vi "MultiAxisPositioningWithTime.vi"(6 "error in":errorcluster, 8 "Input_Cluster":T1, 9 "connection ID":refnum<k5>) -> (0 "error out":errorcluster, 2 "return":T2, 3 "connection ID":refnum<k5>)   [LabVIEW 2016, in "AMC_VIs.lvlib"]
doc: "Simultaneously set 3 axes positions\n and get positions to minimize network latency"
uses:
  AMC_VIs.lvlib
panel:
  out "params_cluster":T3
  in  "Params_cluster":T4
  in  "results_cluster":T5
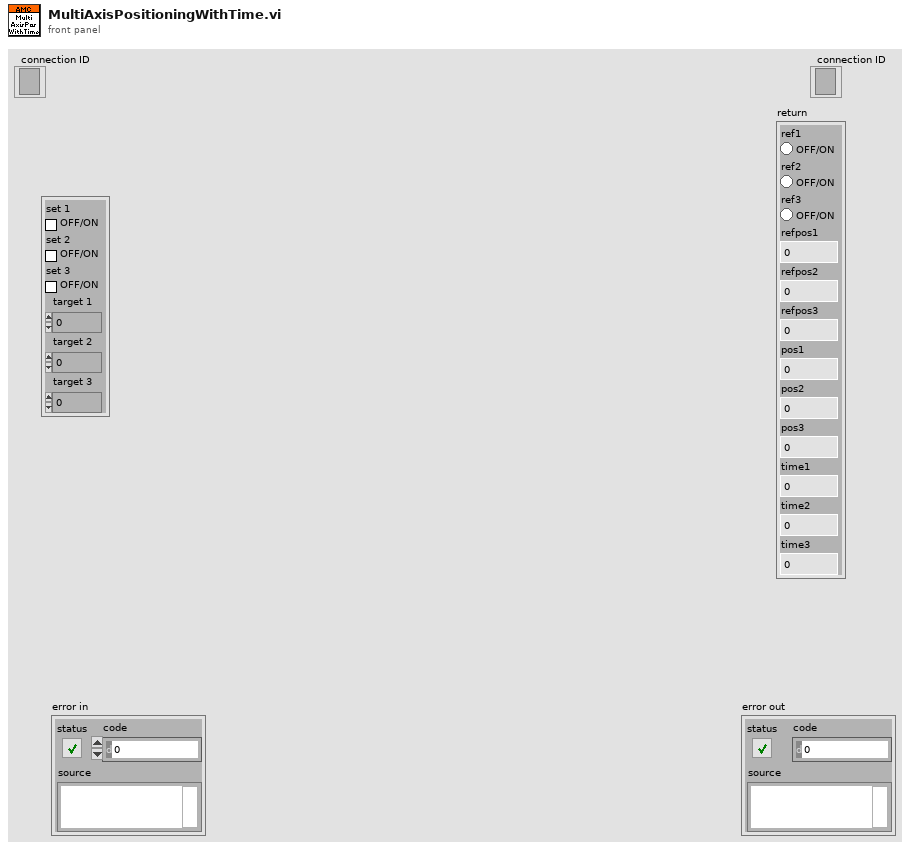
[diagram p1: front panel]
types:
  T1 = cluster{"set 1":bool, "set 2":bool, "set 3":bool, "target 1":i32, "target 2":i32, "target 3":i32}
  T2 = cluster{"ref1":bool, "ref2":bool, "ref3":bool, "refpos1":i32, "refpos2":i32, "refpos3":i32, "pos1":i32, "pos2":i32, "pos3":i32, "time1":dbl, "time2":dbl, "time3":dbl}
  T3 = cluster{"set1":bool, "set2":bool, "set3":bool, "target1":i32, "target2":i32, "target3":i32}
  T4 = cluster{"boolean":bool, "boolean":bool, "boolean":bool, "integer":i32, "integer":i32, "integer":i32}
  T5 = cluster{"errNo":i32, "ref1":bool, "ref2":bool, "ref3":bool, "refpos1":i32, "refpos2":i32, "refpos3":i32, "pos1":i32, "pos2":i32, "pos3":i32, "time1":dbl, "time2":dbl, "time3":dbl}
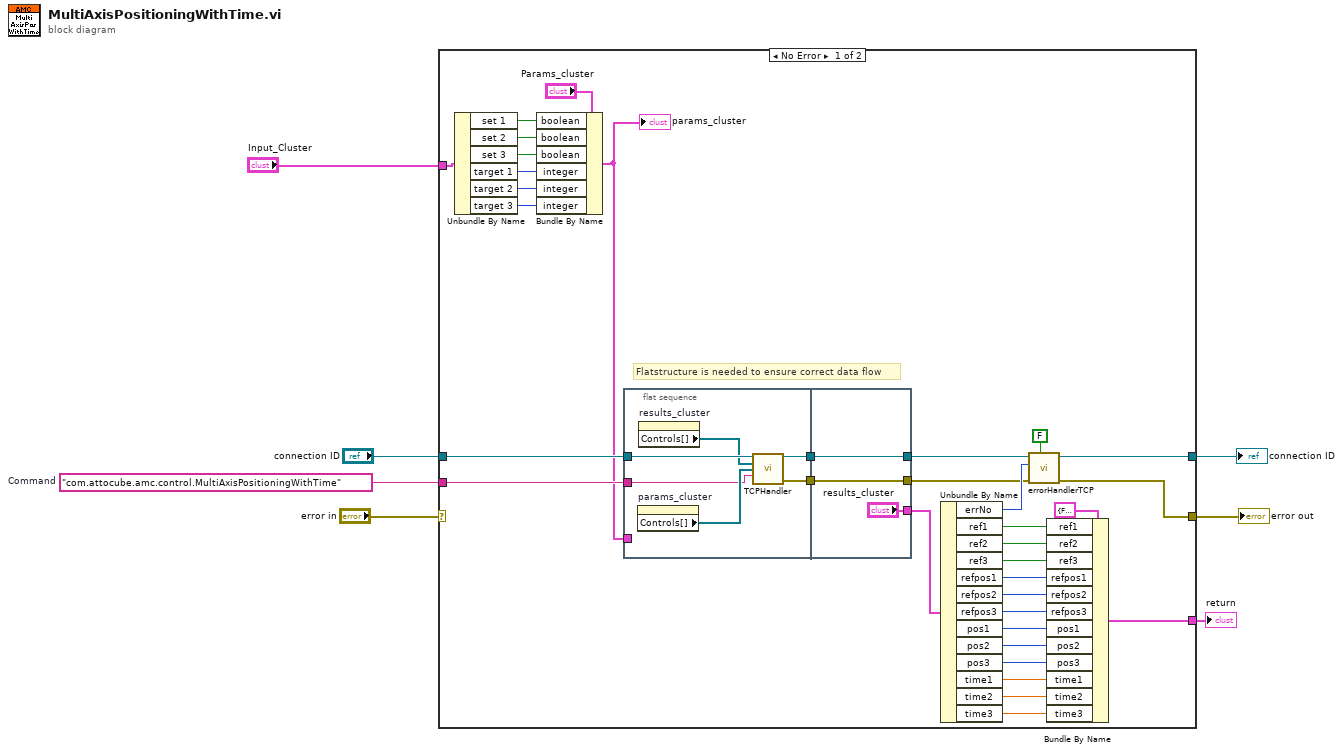
[diagram p0: block diagram]
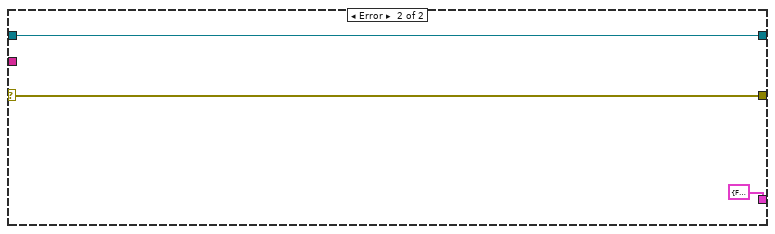
[diagram p2: hidden frame]
diagram:
  w4 = "com.attocube.amc.control.MultiAxisPositioningWithTime"  # Command
  n1 = case shown="No Error" "error in" {
    selector: "error in" -> [_ w52]
    tunnel: [w41 w53] -> w7
    tunnel: "connection ID" -> [w39 w53]
    tunnel: w4 -> [w33 _]
    tunnel: [w16 w52] -> w3
    tunnel: [w15 T2 {"ref1"=FALSE, "ref2"=FALSE, "ref3"=FALSE, "refpos1"=0, "refpos2"=0, "refpos3"=0, "pos1"=0, "pos2"=0, "pos3"=0, "time1"=0.0, "time2"=0.0, "time3"=0.0} ("results_cluster")] -> w2
    tunnel: "Input_Cluster" -> [w14 _]
    frame No Error {
      # "Flatstructure is needed to ensure correct data flow"
      n2 = Unbundle By Name(w14) -> ("set 1"=w13:bool, "set 2"=w12:bool, "set 3"=w11:bool, "target 1"=w10:i32, "target 2"=w9:i32, "target 3"=w8:i32)
      n3 = Bundle By Name(cluster="Params_cluster", "boolean"=w13, "boolean"=w12, "boolean"=w11, "integer"=w10, "integer"=w9, "integer"=w8) -> (w30:T4)
      "params_cluster" <- w30
      n4 = flat-sequence {
        tunnel: [w46] -> w35
        tunnel: w39 -> [w47]
        tunnel: w33 -> [w43]
        tunnel: [w42] -> w31
        tunnel: w30 -> [_]
        tunnel: ["results_cluster"] -> w36
        tunnel: [w50] -> w38
        tunnel: w35 -> [w50]
        tunnel: [w48] -> w32
        tunnel: w31 -> [w48]
        frame #0 {
          n5 = property on="params_cluster" class="Clust (strict)"() -> ("Controls[]"=w44:refnum<vi>[])  [unwired: 2 in, 2 out]
          n6 = property on="results_cluster" class="Clust (strict)"() -> ("Controls[]"=w45:refnum<vi>[])  [unwired: 2 in, 2 out]
          n7 = call "TCPHandler.vi"("connection ID"=w47, "results_cluster"=w45, "params_cluster"=w44, "method"=w43) -> ("connection ID"=w46:refnum<k5>, "error"=w42:errorcluster)  [unwired: 8 in, 2 out]
        }
        frame #1 {
        }
      }
      n8 = Unbundle By Name(w36) -> ("errNo"=w37:i32, "ref1"=w28:bool, "ref2"=w27:bool, "ref3"=w26:bool, "refpos1"=w25:i32, "refpos2"=w24:i32, "refpos3"=w23:i32, "pos1"=w22:i32, "pos2"=w21:i32, "pos3"=w20:i32, "time1"=w19:dbl, "time2"=w18:dbl, "time3"=w17:dbl)
      n9 = call "errorHandlerTCP.vi"("show popup"=FALSE, "error in"=w32, "error number"=w37, "connection ID"=w38) -> ("error out"=w16:errorcluster, "connection ID"=w41:refnum<k5>)  [unwired: 6 in]
      n10 = Bundle By Name(cluster=T2 {"ref1"=FALSE, "ref2"=FALSE, "ref3"=FALSE, "refpos1"=0, "refpos2"=0, "refpos3"=0, "pos1"=0, "pos2"=0, "pos3"=0, "time1"=0.0, "time2"=0.0, "time3"=0.0} ("results_cluster"), "ref1"=w28, "ref2"=w27, "ref3"=w26, "refpos1"=w25, "refpos2"=w24, "refpos3"=w23, "pos1"=w22, "pos2"=w21, "pos3"=w20, "time1"=w19, "time2"=w18, "time3"=w17) -> (w15:T2)
    }
    frame Error {
    }
  }
  "error out" <- w3
  "connection ID" <- w7
  "return" <- w2
